vi "Setup.vi"(0 "Vector Path in":refnum<class "Vector Abstract Path.lvclass">, 11 "error in (no error)":errorcluster) -> (4 "Vector Path out":refnum<class "Vector Abstract Path.lvclass">, 15 "error out":errorcluster)   [LabVIEW 2023, in "RFFixtureCharact.Public.lvlib" / "Vector Abstract Path.lvclass"]
uses:
  Vector Abstract Path.lvclass
  C:/rfcal/AuxTools/STSRFFixtureCharactUtility/Source/Code Modules/Common/Base Classes/Path/Path.lvclass
  Instruments/Cal Standard/Cal Standard Base/Cal Standard Base.lvclass
  Common/Base Classes/Path/Path.lvclass
  Common/RFCalAndFixtureCharact.Common.lvlib
  Instruments/Cal Standard/Cal Standard Factory/Cal Standard Factory.lvclass
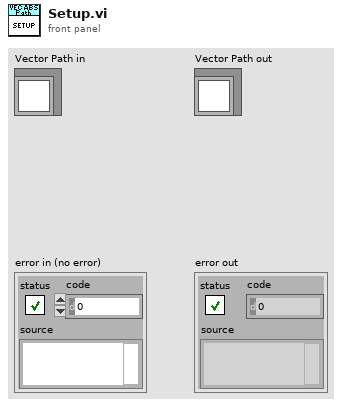
[diagram p1: front panel]
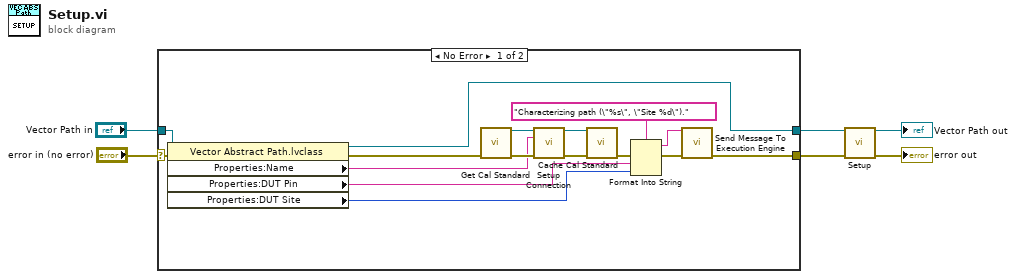
[diagram p0: block diagram]
diagram:
  n1 = case shown="No Error" "error in (no error)" {
    selector: "error in (no error)" -> [w18 w24]
    tunnel: [w15 w24] -> w2
    tunnel: "Vector Path in" -> [w17 w23]
    tunnel: [w8 w23] -> w3
    frame No Error {
      n2 = property class="Vector Abstract Path.lvclass"(reference=w17, error in=w18) -> (reference out=w8:refnum<class "Vector Abstract Path.lvclass">, error out=w7:errorcluster, "Properties:Name"=w9:string, "Properties:DUT Pin"=w16:string, "Properties:DUT Site"=w20:i32)
      n3 = call "Get Cal Standard.vi"("error in (no error)"=w7) -> ("Cal Standard Base out"=w13:refnum<class "Cal Standard Base.lvclass">, "error out"=w14:errorcluster)  [unwired: 12 in, 1 out]
      n4 = call-dynamic "Setup Connection.vi"("Cal Standard Base in"=w13, "Path Name"=w9, "error in (no error)"=w14) -> ("Cal Standard Base out"=w10:refnum<class "Cal Standard Base.lvclass">, "error out"=w12:errorcluster)  [unwired: 11 in]
      n5 = call "Cache Cal Standard.vi"("Cal Standard Base in"=w10, "error in (no error)"=w12) -> ("error out"=w11:errorcluster)  [unwired: 12 in, 1 out]
      n6 = Format Into String(format string="Characterizing path (\"%s\", \"Site %d\")." ("message"), error in=w11, w16, w20) -> (resulting string=w19:string, error out=w21:errorcluster)  [unwired: 1 in]
      n7 = call "Send Message To Execution Engine.vi"("Message"=w19, "error in (no error)"=w21) -> ("error out"=w15:errorcluster)  [unwired: 13 in]
    }
    frame Error {
    }
  }
  n8 = call-parent "Setup.vi"("Path in"=w3, "error in (no error)"=w2) -> ("Path out"=→"Vector Path out":refnum<class "Vector Abstract Path.lvclass">, "error out"=→"error out":errorcluster)  [unwired: 12 in]
